vi "Write Datagram.vi"(5 "destination port":u16, 7 "destination address":u32, 8 "error in (no error)":errorcluster, 9 "timeout ms (25000)":i32=25000 format="%d ms", 10 "data":string, 11 "UDPlog Transceiver in":refnum<class "UDPlog Transceiver.lvclass">) -> (0 "error out":errorcluster, 1 "timed out?":bool, 3 "UDPlog Transceiver out":refnum<class "UDPlog Transceiver.lvclass">)   [LabVIEW 2023, in "UDPlog.lvlib" / "UDPlog Transceiver.lvclass"]
uses:
  UDPlog Transceiver.lvclass
  UDPlog Transceiver.lvclass/UDPlog Transceiver.ctl
  <vilib>/Utility/SystemLogging/NI_SystemLogging.lvlib
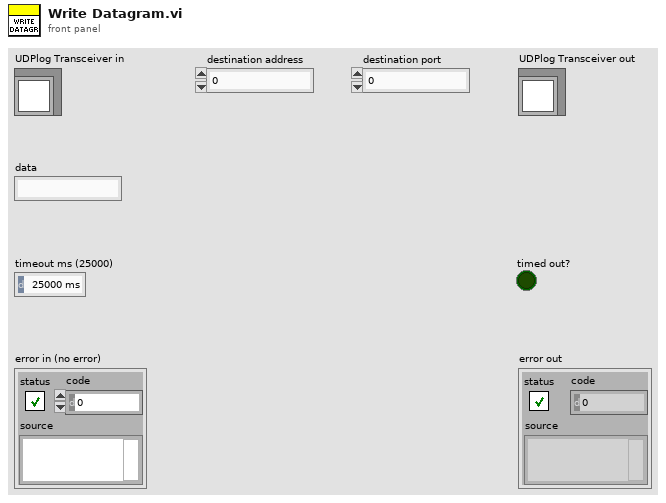
[diagram p1: front panel]
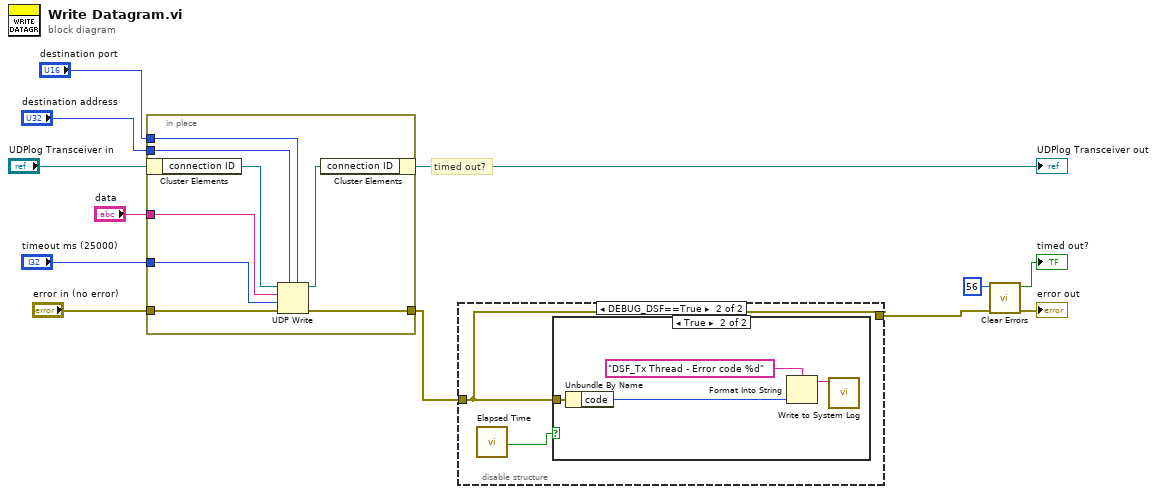
[diagram p0: block diagram]
diagram:
  # "timed out?"
  n1 = in-place {
    in-place-border: "error in (no error)" -> [w20]
    in-place-border: [w19] -> w2
    in-place-border: "timeout ms (25000)" -> [w17]
    in-place-border: "data" -> [w15]
    in-place-border: "destination address" -> [w14]
    in-place-border: "destination port" -> [w13]
    n2 = in-place-cluster #1("UDPlog Transceiver in") -> ("connection ID"=w18:refnum<k16>)
    n3 = UDP Write(address=w14, port or service name=w13, connection ID=w18, data in=w15, 8:w20, 9:w17) -> (error out=w19:errorcluster, 3:w16:refnum<k16>)
    n4 = in-place-cluster #1("connection ID"=w16) -> (→"UDPlog Transceiver out":refnum<class "UDPlog Transceiver.lvclass">)
  }
  n5 = disable-structure shown="DEBUG_DSF==True" {
    disable-tunnel: w2 -> [w21 w23]
    disable-tunnel: [w21 w23] -> w1
    frame condition #0 {
    }
    frame condition #1 (active) {
      n6 = call "Elapsed Time"() -> ("Time has Elapsed"=w22:bool)  [unwired: 12 in, 7 out]
      n7 = case shown="True" w22 {
        tunnel: w23 -> [_ w25]
        frame False {
        }
        frame True {
          n8 = Unbundle By Name(w25) -> ("code"=w24:i32)
          n9 = Format Into String(format string="DSF_Tx Thread - Error code %d", w24) -> (resulting string=w26:string)  [unwired: 2 in, 1 out]
          n10 = call <vilib>:"Write to System Log.vi"("message"=w26) -> ()  [unwired: 10 in, 1 out]
        }
      }
    }
  }
  n11 = call <vilib>:"Clear Errors.vi"("error in (no error)"=w1, "specific error code to clear (0: all)"=56) -> ("error out"=→"error out":errorcluster, "specific error cleared?"=→"timed out?":bool)  [unwired: 4 in]
